vi "Status Temperature Control.vi"(8 "error in (no error)":errorcluster, 11 "heater_parent in":refnum<class "heater_parent.lvclass">) -> (0 "error out":errorcluster, 2 "Heating or cooling on?":bool, 3 "heater_parent out":refnum<class "heater_parent.lvclass">)   [LabVIEW 2020, in "polar_bear_plus_drivers.lvlib" / "heater_parent.lvclass"]
doc: "Check if the heating switch is turned on or not."
uses:
  <instrlib>/RxnRover/Driver Polar Bear Plus/heater_parent/heater_parent.lvclass
  <instrlib>/RxnRover/Driver Polar Bear Plus/heater_parent/heater_parent.lvclass/heater_parent.ctl
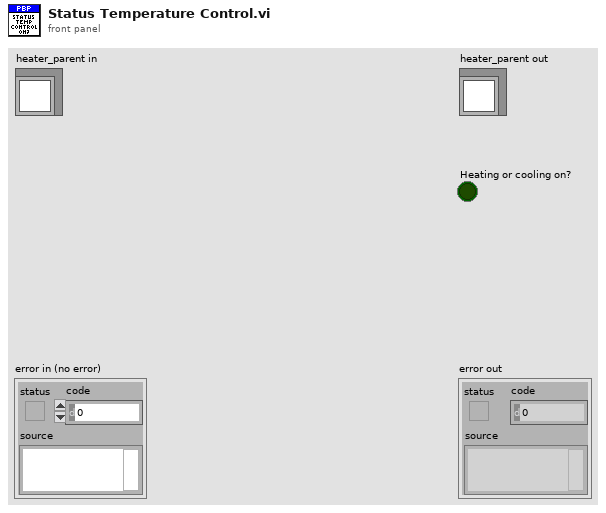
[diagram p1: front panel]
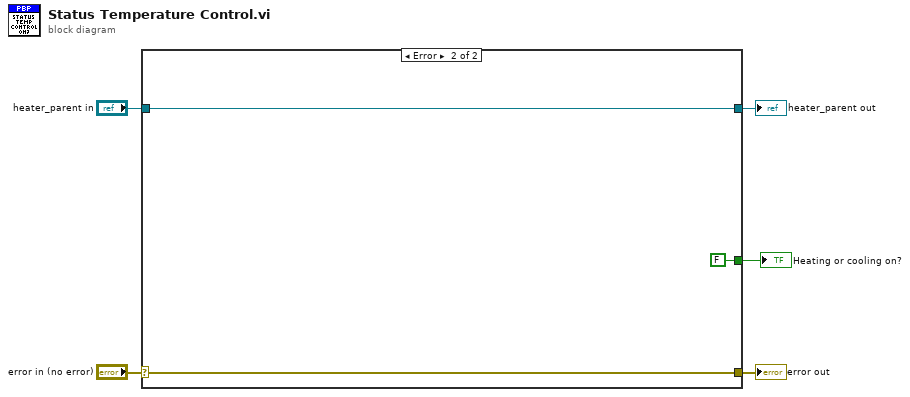
[diagram p0: block diagram]
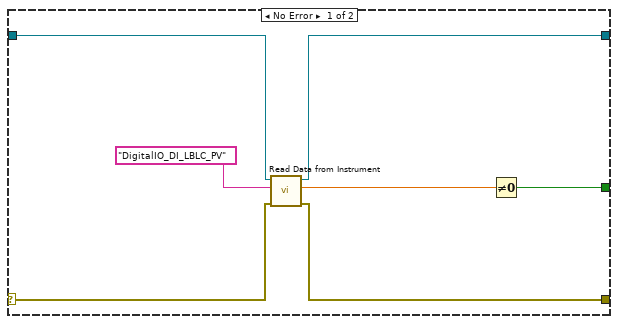
[diagram p2: hidden frame]
diagram:
  n1 = case shown="Error" "error in (no error)" {
    selector: "error in (no error)" -> [w11 w15]
    tunnel: [w10 w15] -> w4
    tunnel: [w9 w14] -> w2
    tunnel: "heater_parent in" -> [w12 w14]
    tunnel: [w6 FALSE] -> w1
    frame No Error {
      n2 = call-dynamic "Read Data from Instrument.vi"("error in (no error)"=w11, "Address"="DigitalIO_DI_LBLC_PV", "heater_parent in"=w12) -> ("error out"=w10:errorcluster, "Value Read"=w7:dbl, "heater_parent out"=w9:refnum<class "heater_parent.lvclass">)  [unwired: 6 in]
      n3 = Not Equal To 0?(x=w7) -> (x != 0?=w6:bool)
    }
    frame Error {
    }
  }
  "error out" <- w4
  "heater_parent out" <- w2
  "Heating or cooling on?" <- w1
